vi "PV Digiline relay switch point.vi"(8 "error in (no error)":errorcluster, 9 "DigiLine-Cluster":T1={"Parameter"=0, "Parameter\nread only<->describe"=FALSE, "Pressure switch point (mbar)"=1.0} {"Pressure switch point (mbar)" min=5e-10 max=2000.0 step=1.0 format="%_3e"; "Parameter" items=[" Pressure Set Point 1 [hPa ; mbar]", " Pressure Set Point 2 [hPa ; mbar]"]}, 10 "Adress of unit":u16=1 max=999 step=1, 11 "VISA session":refnum<visa-resource-name>) -> (0 "error out":errorcluster, 2 "response (data)":string, 3 "dup VISA session":refnum<visa-resource-name>)   [LabVIEW 2021, in "Pfeiffer Vacuum.lvlib"]
doc: "There are tow parameters available, only one of which can be enabled at a time. \n\n0 - Pressure switch point 1 [mbar] (default)\n1 - Pressure switch point 2 [mbar] \n\nNote: The one control right of this one will set the appropriate values for the selected parameter. Any settings for an parameter that is not selected will be ignored. If a value is out of range, it will be changed to either the upper or the lower limit of the range."
uses:
  <instrlib>/Pfeiffer Vacuum/Pfeiffer Vacuum.lvlib
  <instrlib>/Pfeiffer Vacuum/Public/DigiLine/PV Digiline relay switch point - Cluster.ctl
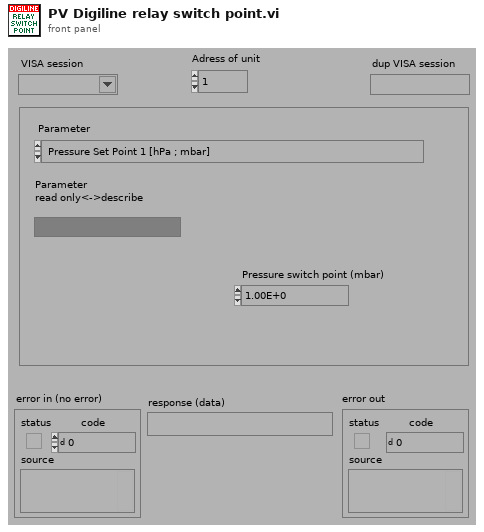
[diagram p1: front panel]
types:
  T1 = typedef "Pfeiffer Vacuum.lvlib/PV Digiline relay switch point - Cluster.ctl" = cluster{"Parameter":u16, "Parameter\nread only<->describe":bool, "Pressure switch point (mbar)":dbl}
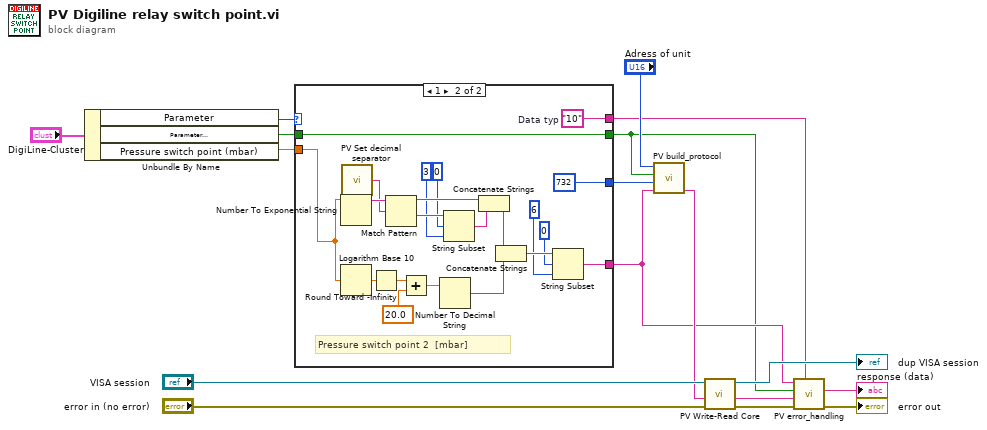
[diagram p0: block diagram]
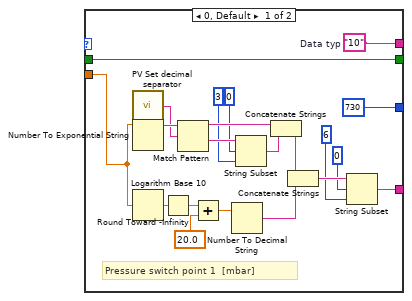
[diagram p2: hidden frame]
diagram:
  n1 = Unbundle By Name("DigiLine-Cluster") -> ("Parameter"=w14:u16, "Parameter\nread only<->describe"=w13:bool, "Pressure switch point (mbar)"=w1:dbl)
  n2 = case shown="1" w14 {
    tunnel: [u16 730 ("Parameter-number") u16 732 ("Parameter-number")] -> w16
    tunnel: [w19 w40] -> w4
    tunnel: [w37 w58] -> w3
    tunnel: w13 -> [w37 w58]
    tunnel: w1 -> [w20 w41]
    tunnel: [w36 w57] -> w5
    frame 0, Default {
      w36 = "10"  # Data typ
      # "Pressure switch point 1  [mbar]"
      n3 = call <instrlib>:"PV Set decimal separator.vi"() -> ("decimal separator"=w18:string)
      n4 = Number To Exponential String(number=w20) -> (E-format string=w32:string)  [unwired: 3 in]
      n5 = Logarithm Base 10(1:w20) -> (0:w35:dbl)
      n6 = Round Toward -Infinity(1:w35) -> (0:w34:dbl)
      n7 = Match Pattern(string=w32, regular expression=w18) -> (before substring=w33:string, after substring=w31:string)  [unwired: 1 in, 2 out]
      n8 = Add(x=w34, y=20.0) -> (x+y=w27:dbl)
      n9 = Number To Decimal String(number=w27) -> (decimal integer string=w24:string)  [unwired: 1 in]
      n10 = String Subset(string=w31, offset (0)=0 ("Offset (0)"), length (rest)=3 ("Länge")) -> (substring=w28:string)
      n11 = Concatenate Strings(w33, w28) -> (w25:string)
      n12 = Concatenate Strings(w25, w24) -> (w23:string)
      n13 = String Subset(string=w23, offset (0)=0 ("Offset (0)"), length (rest)=6 ("Länge")) -> (substring=w19:string)
    }
    frame 1 {
      w57 = "10"  # Data typ
      # "Pressure switch point 2  [mbar]"
      n14 = Number To Exponential String(number=w41) -> (E-format string=w53:string)  [unwired: 3 in]
      n15 = Logarithm Base 10(1:w41) -> (0:w56:dbl)
      n16 = call <instrlib>:"PV Set decimal separator.vi"() -> ("decimal separator"=w39:string)
      n17 = Round Toward -Infinity(1:w56) -> (0:w55:dbl)
      n18 = Match Pattern(string=w53, regular expression=w39) -> (before substring=w54:string, after substring=w52:string)  [unwired: 1 in, 2 out]
      n19 = Add(x=w55, y=20.0) -> (x+y=w48:dbl)
      n20 = Number To Decimal String(number=w48) -> (decimal integer string=w45:string)  [unwired: 1 in]
      n21 = String Subset(string=w52, offset (0)=0 ("Offset (0)"), length (rest)=3 ("Länge")) -> (substring=w49:string)
      n22 = Concatenate Strings(w54, w49) -> (w46:string)
      n23 = Concatenate Strings(w46, w45) -> (w44:string)
      n24 = String Subset(string=w44, offset (0)=0 ("Offset (0)"), length (rest)=6 ("Länge")) -> (substring=w40:string)
    }
  }
  n25 = call <instrlib>:"PV build_protocol.vi"("Data"=w4, "Parameter-number"=w16, "parameter\nread<->describe"=w3, "Adress"="Adress of unit") -> ("output"=w9:string)  [unwired: 3 in]
  n26 = call <instrlib>:"PV Write-Read Core.vi"("error in"="error in (no error)", "Write data in"=w9, "VISA session"="VISA session") -> ("error out"=w6:errorcluster, "response (data) out"=w7:string, "dup VISA session"=→"dup VISA session":refnum<visa-resource-name>)  [unwired: 2 in]
  n27 = call <instrlib>:"PV error_handling.vi"("Data Typ in"=w5, "error in"=w6, "response (data) in"=w7, "Parameter\nread only<->describe"=w3, "data in"=w4) -> ("error out"=→"error out":errorcluster, "Data out"=→"response (data)":string)  [unwired: 4 in, 1 out]
